vi "status.vi"(8 "error IO":errorcluster, 11 "enable":bool[](array[boolean])) -> (0 "error out":errorcluster, 2 "Actual Positions":i32[](array[numeric]), 3 "stopped?":bool[](array[boolean]))   [LabVIEW 2013, in "PicoMotor.lvclass"]
uses:
  PicoMotor.lvclass
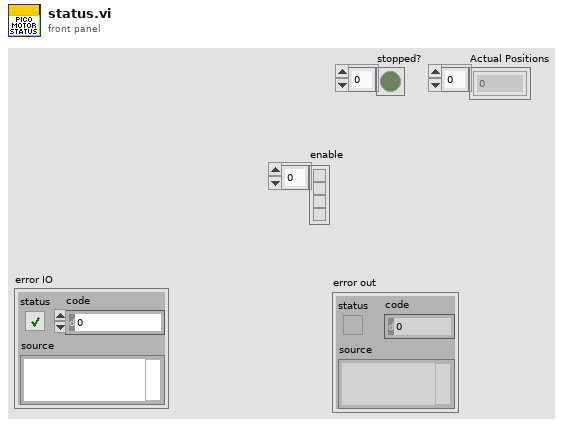
[diagram p1: front panel]
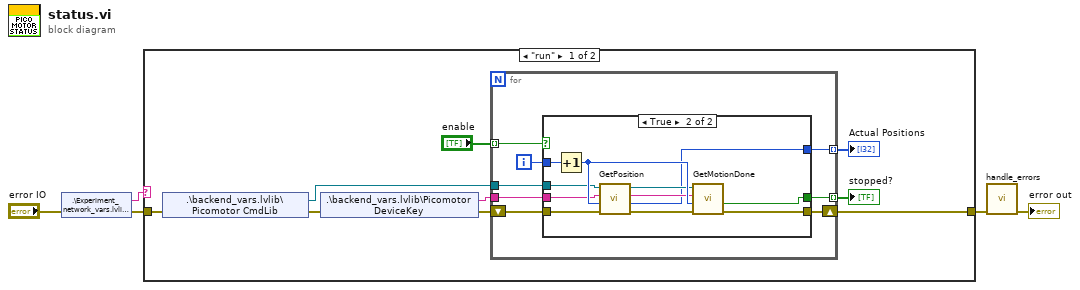
[diagram p0: block diagram]
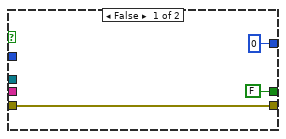
[diagram p2: hidden frame]
diagram:
  n1 = shared-variable ".\\Experiment_network_vars.lvlib\\state"(error in="error IO") -> (w3:string, error out=w1:errorcluster)
  n2 = case shown="\"run\"" w3 {
    tunnel: [w14 w37] -> w5
    tunnel: w1 -> [w11 w37]
    frame "run" {
      n3 = shared-variable ".\\backend_vars.lvlib\\Picomotor CmdLib"(error in=w11) -> (w12:refnum<k24>, error out=w10:errorcluster)
      n4 = shared-variable ".\\backend_vars.lvlib\\Picomotor DeviceKey"(error in=w10) -> (w13:string, error out=w6:errorcluster)
      n5 = for {
        shift-right: [w18] -> w14
        shift-left: w6 -> [w21]
        tunnel: w13 -> [w20]
        tunnel: w12 -> [w19]
        tunnel: [w17] -> w9 mode=indexing
        tunnel: [w16] -> w8 mode=indexing
        tunnel: "enable" -> [w15] mode=indexing
        i -> [w22]
        n6 = case shown="True" w15 {
          tunnel: w22 -> [_ w36]
          tunnel: w21 -> [w25 w28]
          tunnel: w20 -> [_ w29]
          tunnel: w19 -> [_ w30]
          tunnel: [w25 w31] -> w18
          tunnel: [FALSE ("Is Motion Done") w27] -> w17
          tunnel: [0 ("Position") w26] -> w16
          frame False {
          }
          frame True {
            n7 = Increment(x=w36) -> (x+1=w34:i32)
            n8 = call "GetPosition.vi"("error in (no error)"=w28, "Motor"=w34, "DeviceKey In"=w29, "CmdLib In"=w30) -> ("error out"=w35:errorcluster, "Position"=w26:i32, "DeviceKey Out"=w32:string, "CmdLib Out"=w33:refnum<k24>)
            n9 = call "GetMotionDone.vi"("error in (no error)"=w35, "Motor"=w34, "DeviceKey In"=w32, "CmdLib In"=w33) -> ("error out"=w31:errorcluster, "Is Motion Done"=w27:bool)  [unwired: 2 out]
          }
        }
      }
      "stopped?" <- w9
      "Actual Positions" <- w8
    }
    frame "halt", Default {
    }
  }
  n10 = call "handle_errors.vi"("error in (no error)"=w5) -> ("error out"=→"error out":errorcluster)  [unwired: 10 in]
